vi "K_matrix.vi"(0 "new_P22":fxp<+,32,16>, 1 "output valid":bool, 2 "P22_new":fxp<+,32,16>, 3 "new_P11":fxp<+,32,16>, 4 "output valid 2":bool, 6 "P31_new":fxp<+,32,16>, 7 "P42_new":fxp<+,32,16>, 8 "var_x":fxp<+,16,4>, 9 "var_y":fxp<+,16,4>, 11 "P11_new":fxp<+,32,16>) -> (10 "output valid 11":bool, 12 "K11":fxp<+,32,16>, 13 "output valid 22":bool, 14 "K31":fxp<+,32,16>, 15 "output valid 31":bool, 16 "K42":fxp<+,32,16>, 17 "output valid 42":bool, 18 "K22":fxp<+,32,16>)   [LabVIEW 2020]
uses:
  <vilib>/rvi/FXPMathLib/FxpDiv/subVIs/nifxpmath_Div_SimConfig.ctl
  <vilib>/rvi/FXPMathLib/FxpDiv/simVIs/DllFxpDivTemp_sub.vi
  <vilib>/rvi/FXPMathLib/FxpDiv/XNode/nifxpmath_Div.xnode
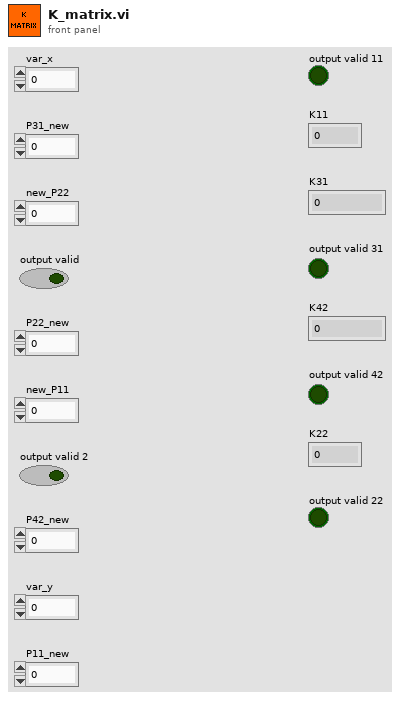
[diagram p1: front panel]
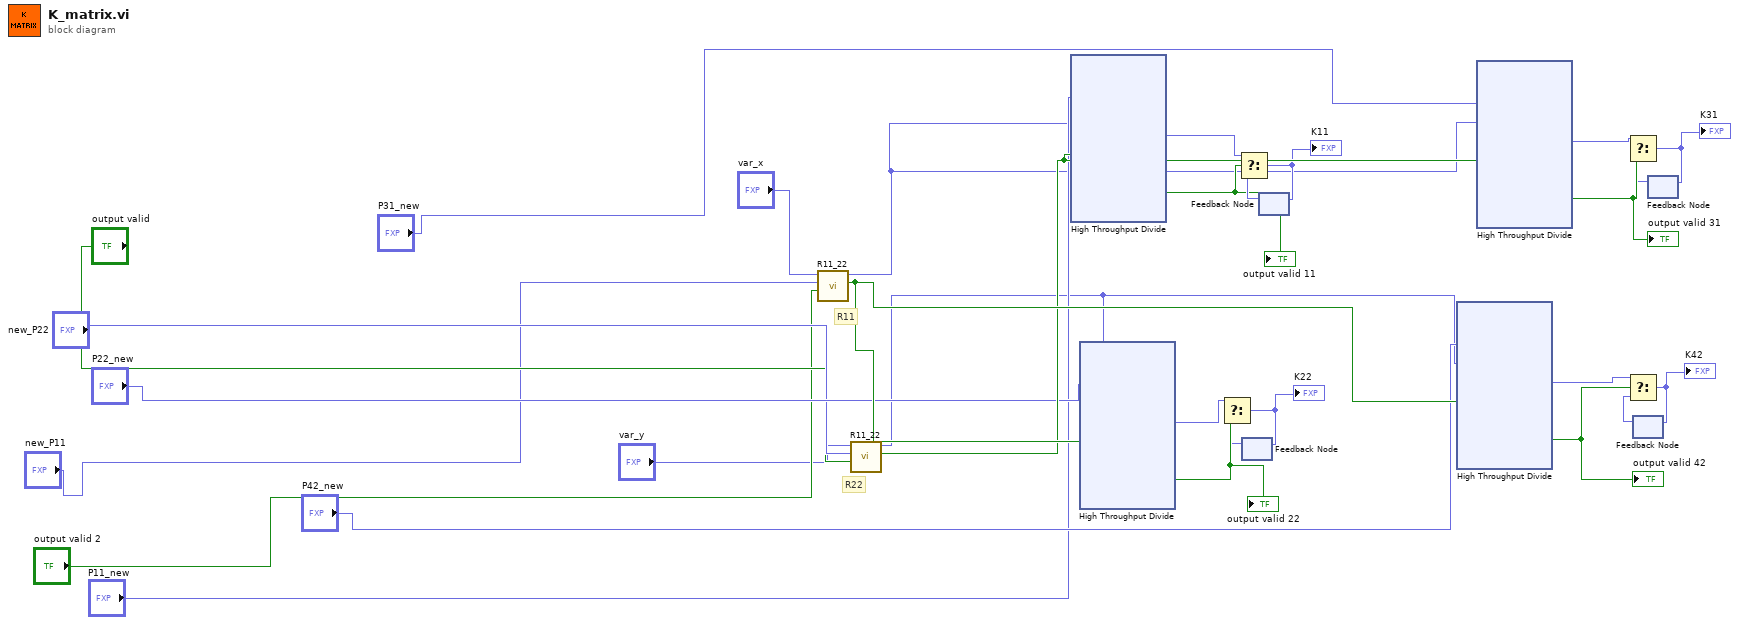
[diagram p0: block diagram]
diagram:
  # "R11"
  # "R22"
  n1 = call "R11_22.vi"("output valid in"="output valid 2", "new_P11"="new_P11", "var_x"="var_x") -> ("output valid out"=w26:bool, "R11"=w1:fxp<+,32,16>)  [unwired: 7 in]
  n2 = call "R11_22.vi"("output valid in"="output valid", "new_P11"="new_P22", "var_x"="var_y") -> ("output valid out"=w20:bool, "R11"=w2:fxp<+,32,16>)  [unwired: 7 in]
  n3 = xnode "High Throughput Divide"("x"="P11_new", "y"=w1, "input valid"=w20) -> ("x/y"=w11:fxp<+,32,16>, "output valid"=w10:bool)  [unwired: 1 in, 1 out]
  "output valid 11" <- w10
  n4 = xnode "High Throughput Divide"("x"="P22_new", "y"=w2, "input valid"=w26) -> ("x/y"=w17:fxp<+,32,16>, "output valid"=w18:bool)  [unwired: 1 in, 1 out]
  "output valid 22" <- w18
  n5 = feedback #1() -> (w16:fxp<+,32,16>)  [unwired: 1 in]
  n6 = Select(t=w17, s=w18, f=w16) -> (s? t:f=w15:fxp<+,32,16>)
  "K22" <- w15
  n7 = feedback-in #1(w15) -> ()
  n8 = feedback #2() -> (w13:fxp<+,32,16>)  [unwired: 1 in]
  n9 = Select(t=w11, s=w10, f=w13) -> (s? t:f=w12:fxp<+,32,16>)
  "K11" <- w12
  n10 = feedback-in #2(w12) -> ()
  n11 = xnode "High Throughput Divide"("x"="P42_new", "y"=w2, "input valid"=w26) -> ("x/y"=w29:fxp<+,32,16>, "output valid"=w28:bool)  [unwired: 1 in, 1 out]
  "output valid 42" <- w28
  n12 = xnode "High Throughput Divide"("x"="P31_new", "y"=w1, "input valid"=w20) -> ("x/y"=w23:fxp<+,32,16>, "output valid"=w24:bool)  [unwired: 1 in, 1 out]
  "output valid 31" <- w24
  n13 = feedback #3() -> (w30:fxp<+,32,16>)  [unwired: 1 in]
  n14 = Select(t=w29, s=w28, f=w30) -> (s? t:f=w27:fxp<+,32,16>)
  "K42" <- w27
  n15 = feedback-in #3(w27) -> ()
  n16 = feedback #4() -> (w22:fxp<+,32,16>)  [unwired: 1 in]
  n17 = Select(t=w23, s=w24, f=w22) -> (s? t:f=w21:fxp<+,32,16>)
  "K31" <- w21
  n18 = feedback-in #4(w21) -> ()
